vi "Configure Arbitrary Waveform (Current).vi"(5 "Repeat Continuously (False)":bool, 6 "Terminate Option (0: Original Value)":u16(ring) items=["Original Value", "Last Value"], 7 "Count (1)":u16=1, 8 "error in (no error)":errorcluster, 9 "Dwell Time (0.001)":dbl=0.001, 10 "Current Points  (Blank)":dbl[](array[numeric]), 11 "VISA resource name":refnum<visa-resource-name>) -> (0 "error out":errorcluster, 3 "VISA resource name out":refnum<visa-resource-name>)   [LabVIEW 2019, in "Agilent N7976A.lvlib"]
doc: "Configures the arbitrary current waveform with information regarding the dwell time, the repeat settings, the termination settings and the values of the current values."
uses:
  <instrlib>/Agilent N7976A/Agilent N7976A.lvlib
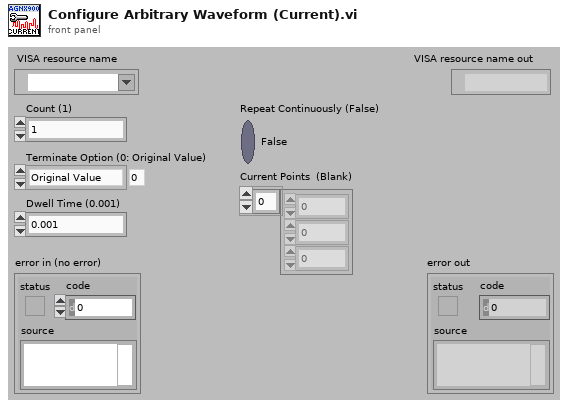
[diagram p1: front panel]
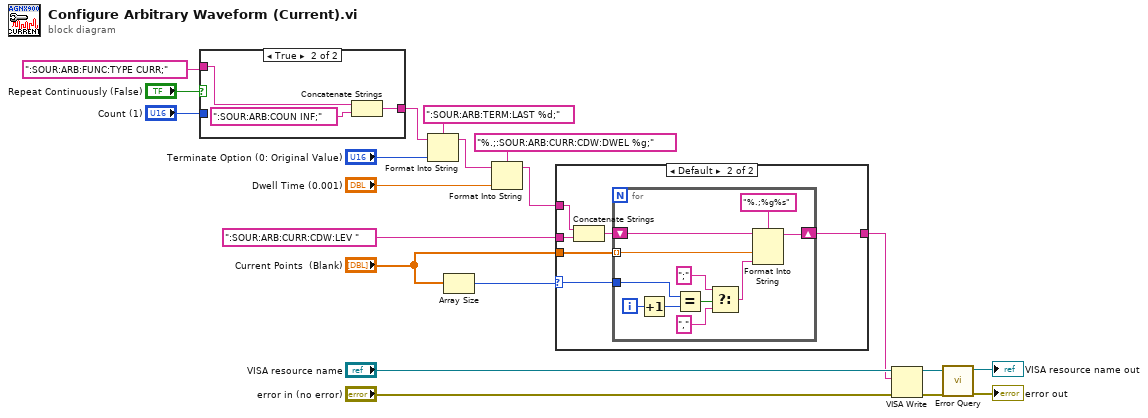
[diagram p0: block diagram]
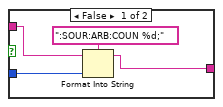
[diagram p2: hidden frame]
diagram:
  n1 = case shown="True" "Repeat Continuously (False)" {
    tunnel: "Count (1)" -> [w23 _]
    tunnel: ":SOUR:ARB:FUNC:TYPE CURR;" -> [w21 w27]
    tunnel: [w22 w25] -> w1
    frame False {
      n2 = Format Into String(format string=":SOUR:ARB:COUN %d;", initial string=w21, w23) -> (resulting string=w22:string)  [unwired: 1 in, 1 out]
    }
    frame True {
      n3 = Concatenate Strings(w27, ":SOUR:ARB:COUN INF;" ("string")) -> (w25:string)
    }
  }
  n4 = Format Into String(format string=":SOUR:ARB:TERM:LAST %d;", initial string=w1, "Terminate Option (0: Original Value)") -> (resulting string=w7:string)  [unwired: 1 in, 1 out]
  n5 = Array Size(array="Current Points  (Blank)") -> (size(s)=w13:i32)
  n6 = Format Into String(format string="%.;:SOUR:ARB:CURR:CDW:DWEL %g;", initial string=w7, "Dwell Time (0.001)") -> (resulting string=w10:string)  [unwired: 1 in, 1 out]
  n7 = case shown="Default" w13 {
    selector: w13 -> [_ w33]
    tunnel: ":SOUR:ARB:CURR:CDW:LEV " -> [_ w31]
    tunnel: "Current Points  (Blank)" -> [_ w34]
    tunnel: w10 -> [w28 w30]
    tunnel: [w28 w29] -> w14
    frame 0 {
    }
    frame Default {
      n8 = Concatenate Strings(w30, w31) -> (w32:string)
      n9 = for {
        tunnel: w34 -> [w44] mode=indexing
        shift-right: [w35] -> w29
        shift-left: w32 -> [w45]
        tunnel: w33 -> [w40]
        i -> [w42]
        n10 = Increment(x=w42) -> (x+1=w41:i32)
        n11 = Equal?(x=w40, y=w41) -> (x = y?=w39:bool)
        n12 = Select(t=";", s=w39, f=",") -> (s? t:f=w36:string)
        n13 = Format Into String(format string="%.;%g%s", initial string=w45, w44, w36) -> (resulting string=w35:string)  [unwired: 1 in, 1 out]
      }
    }
  }
  n14 = VISA Write(VISA resource name="VISA resource name", write buffer=w14, error in (no error)="error in (no error)") -> (VISA resource name out=w17:refnum<visa-resource-name>, error out=w18:errorcluster)  [unwired: 1 out]
  n15 = call <instrlib>:"Error Query.vi"("error in (no error)"=w18, "VISA resource name"=w17) -> ("error out"=→"error out":errorcluster, "VISA resource name out"=→"VISA resource name out":refnum<visa-resource-name>)  [unwired: 6 in, 2 out]
